vi "Initialize.vi"(8 "error in (no error)":errorcluster, 11 "TCS in":refnum<class "TCS.lvclass">) -> (0 "error out":errorcluster, 3 "TCS out":refnum<class "TCS.lvclass">)   [LabVIEW 2018, in "TCS.lvclass"]
uses:
  TCS.lvclass
  Server/Server.lvclass
  Comm/Stream/Stream.lvclass
  Log/Log.lvclass
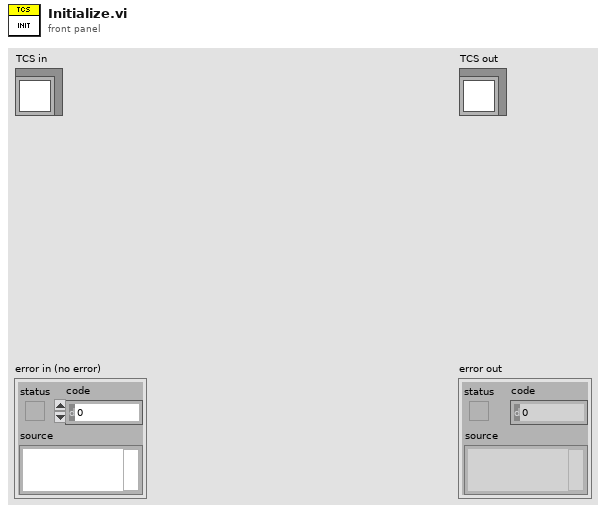
[diagram p1: front panel]
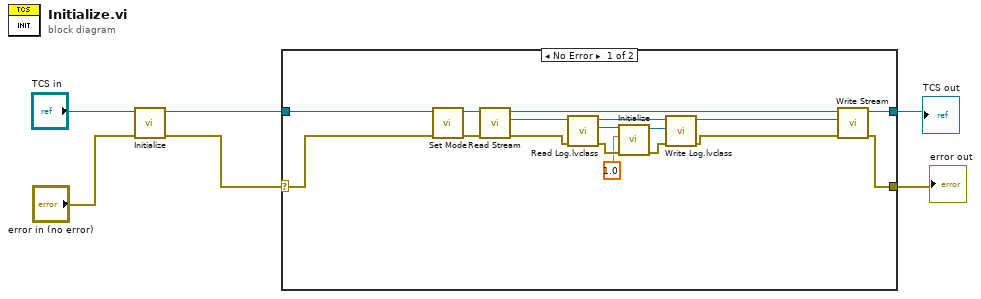
[diagram p0: block diagram]
diagram:
  n1 = call-parent "Initialize.vi"("error in (no error)"="error in (no error)", "Server in"="TCS in") -> ("error out"=w4:errorcluster, "Server out"=w3:refnum<class "TCS.lvclass">)  [unwired: 8 in]
  n2 = case shown="No Error" w4 {
    selector: w4 -> [w9 w24]
    tunnel: w3 -> [w10 w25]
    tunnel: [w22 w25] -> w1
    tunnel: [w21 w24] -> w2
    frame No Error {
      n3 = call-dynamic "Set Mode.vi"("error in (no error)"=w9, "TCS in"=w10) -> ("error out"=w11:errorcluster, "TCS out"=w12:refnum<class "TCS.lvclass">)  [unwired: 8 in]
      n4 = call-dynamic "Read Stream.vi"("error in (no error)"=w11, "Server in"=w12) -> ("error out"=w7:errorcluster, "Stream.lvclass"=w8:refnum<class "Stream.lvclass">, "Server out"=w23:refnum<class "TCS.lvclass">)  [unwired: 7 in]
      n5 = call-dynamic "Read Log.lvclass.vi"("error in (no error)"=w7, "Comm in"=w8) -> ("error out"=w17:errorcluster, "Log.lvclass"=w19:refnum<class "Log.lvclass">, "Comm out"=w20:refnum<class "Stream.lvclass">)  [unwired: 7 in]
      n6 = call-dynamic "Initialize.vi"("error in (no error)"=w17, "Level"=1.0, "Log in"=w19) -> ("error out"=w16:errorcluster, "Log out"=w18:refnum<class "Log.lvclass">)  [unwired: 7 in]
      n7 = call-dynamic "Write Log.lvclass.vi"("error in (no error)"=w16, "Log.lvclass"=w18, "Comm in"=w20) -> ("error out"=w14:errorcluster, "Comm out"=w15:refnum<class "Stream.lvclass">)  [unwired: 7 in]
      n8 = call-dynamic "Write Stream.vi"("error in (no error)"=w14, "Stream.lvclass"=w15, "Server in"=w23) -> ("error out"=w21:errorcluster, "Server out"=w22:refnum<class "TCS.lvclass">)  [unwired: 7 in]
    }
    frame Error {
    }
  }
  "error out" <- w2
  "TCS out" <- w1
